vi "SOC_calculator (SubVI) RT.vi"(3 "Pre SOC ( / )":dbl=1.0, 4 "capacity usable(Ah)":dbl, 5 "Current(A)":dbl, 6 "tf integral (ms)":i32) -> (0 "Actual SOC( / )":dbl, 1 "SOC(%)":dbl, 2 "resolucion  \nSOC % / 1s":dbl)   [LabVIEW 2017]
uses:
  <vilib>/Analysis/NI_AALPro.lvlib
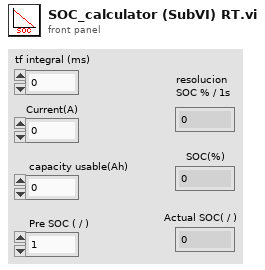
[diagram p1: front panel]
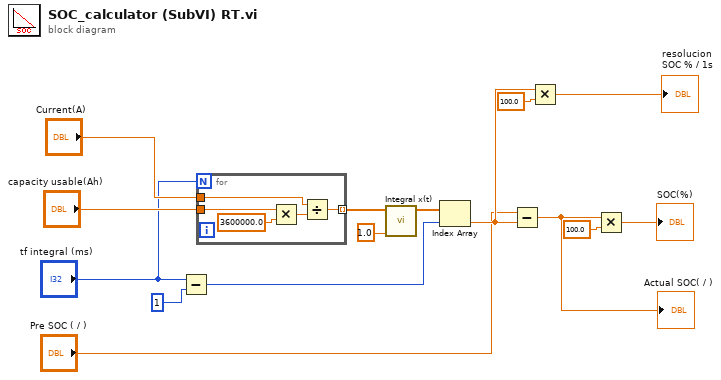
[diagram p0: block diagram]
diagram:
  n1 = Subtract(x="tf integral (ms)", y=1) -> (x-y=w2:i32)
  n2 = for {
    N: "tf integral (ms)" -> [_]
    tunnel: "capacity usable(Ah)" -> [w20]
    tunnel: "Current(A)" -> [w17]
    tunnel: [w18] -> w12 mode=indexing
    n3 = Multiply(x=w20, y=3600000.0) -> (x*y=w19:dbl)
    n4 = Divide(x=w17, y=w19) -> (x/y=w18:dbl)
  }
  n5 = call <vilib>:"Integral x(t).vi"("dt"=1.0, "X"=w12) -> ("Integral X"=w11:dbl[])  [unwired: 8 in, 1 out]
  n6 = Index Array(array=w11, index=w2) -> (element=w15:dbl)
  n7 = Subtract(x="Pre SOC ( / )", y=w15) -> (x-y=w7:dbl)
  "Actual SOC( / )" <- w7
  n8 = Multiply(x=w15, y=100.0) -> (x*y=→"resolucion  \nSOC % / 1s":dbl)
  n9 = Multiply(x=w7, y=100.0) -> (x*y=→"SOC(%)":dbl)
